vi "convertUMLModelXMIToSALXML.vi"(4 "For LabVIEW":bool=TRUE, 6 "Skip enumerations with duplicate values":bool, 7 "Environment options":T2={"Python script file"=path "/home/plotz/Desktop/GeneratedXMLs/UMLToSALXML-MD.py", "SAL Version"="3.7.2"}, 8 "error in (no error)":errorcluster, 9 "Source and Destination Paths":T1={"Source UML XMI file"=path "/home/plotz/Desktop/GeneratedXMLs/ATAOS.xml", "Destination Parent SAL XML directory"=path "/home/plotz/Desktop/GeneratedXMLs"}, 10 "Component Name":string="AtAOS") -> (0 "error out":errorcluster)   [LabVIEW 2016]
uses:
  Typedefs/EnvironmentOptions.ctl
  Typedefs/SourceAndDestinationPaths.ctl
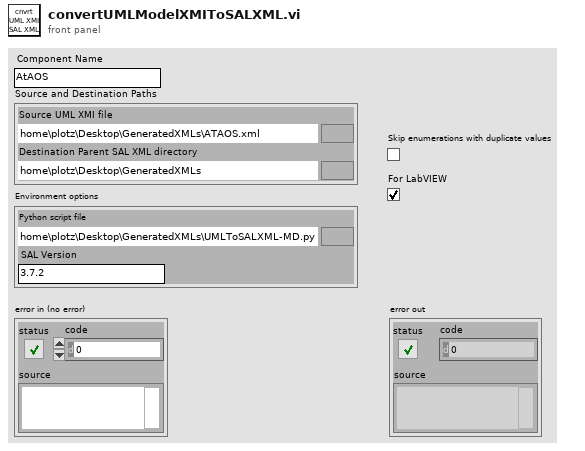
[diagram p1: front panel]
types:
  T1 = typedef "SourceAndDestinationPaths.ctl" = cluster{"Source UML XMI file":path, "Destination Parent SAL XML directory":path}
  T2 = typedef "EnvironmentOptions.ctl" = cluster{"Python script file":path, "SAL Version":string}
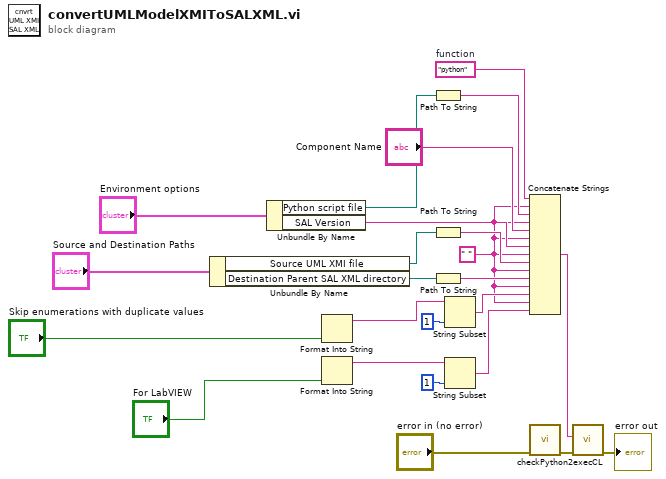
[diagram p0: block diagram]
diagram:
  w3 = " " ("string")
  w24 = "python"  # function
  n1 = Unbundle By Name("Source and Destination Paths") -> ("Source UML XMI file"=w17:path, "Destination Parent SAL XML directory"=w15:path)
  n2 = Unbundle By Name("Environment options") -> ("Python script file"=w21:path, "SAL Version"=w18:string)
  n3 = Format Into String("Skip enumerations with duplicate values") -> (resulting string=w9:string)  [unwired: 3 in, 1 out]
  n4 = Format Into String("For LabVIEW") -> (resulting string=w6:string)  [unwired: 3 in, 1 out]
  n5 = Path To String(path=w21) -> (string=w20:string)
  n6 = Path To String(path=w17) -> (string=w16:string)
  n7 = Path To String(path=w15) -> (string=w14:string)
  n8 = String Subset(string=w9, length (rest)=1 ("length (rest)")) -> (substring=w5:string)  [unwired: 1 in]
  n9 = String Subset(string=w6, length (rest)=1 ("length (rest)")) -> (substring=w4:string)  [unwired: 1 in]
  n10 = Concatenate Strings(w24, w3, w20, w3, "Component Name", w3, w18, w3, w16, w3, w14, w3, w5, w3, w4) -> (w11:string)
  n11 = call "checkPython2.vi"("error in (no error)"="error in (no error)") -> ("error out"=w1:errorcluster)  [unwired: 10 in]
  n12 = call "execCL.vi"("error in (no error)"=w1, "command line"=w11) -> ("error out"=→"error out":errorcluster)  [unwired: 6 in, 3 out]
